vi "HFRR ADV v01.vi"() -> ()   [LabVIEW 2025] (continued)
      frame "Custom" {
      }
    }
    n2158 = Or(x=w2405, y=w2403) -> (x .or. y?=w2404:bool)
    n2159 = case shown="\"About\"" w2402 {
      tunnel: [T29."Acquire" ("Main Tab") T29."Compare Files" ("Main Tab") T29."About" ("Main Tab")] -> w2413
      frame "Acquire", Default {
      }
      frame "Compare Files" {
      }
      frame "About" {
      }
    }
    n2160 = Or(x=w2408, y="OPEN") -> (x .or. y?=w2409:bool)
    n2161 = case shown="True" w2409 {
      tunnel: w2408 -> [_ w2441]
      frame False {
      }
      frame True {
        n2162 = stacked-sequence {
          tunnel: w2441 -> [_ w2508 _ _]
          frame #0 {
            w2457 = "  " ("String 6")
            n2163 = local write "OPEN"(FALSE ("open")) -> ()
            n2164 = local read "string1 2"() -> (w2445:string)
            n2165 = local read "string1 3"() -> (w2444:string)
            n2166 = local read "string1 4"() -> (w2443:string)
            n2167 = property on="OPEN" class="Bool (strict)"("Visible"=FALSE) -> ()  [unwired: 2 in, 2 out]
            n2168 = local write "String 6"(w2457) -> ()
            n2169 = local write "String 7"(w2457) -> ()
            n2170 = local write "String 8"(w2457) -> ()
            n2171 = local write "String 12"(w2457) -> ()
            n2172 = local read "OK Button 16"() -> (w2442:bool)
            n2173 = String To Path(string=w2445) -> (path=w2453:path)
            n2174 = String To Path(string=w2444) -> (path=w2452:path)
            n2175 = String To Path(string=w2443) -> (path=w2451:path)
            n2176 = case shown="True" w2442 {
              tunnel: [w2458 w2459] -> w2446
              frame False {
                n2177 = local read "string1"() -> (w2458:string)
              }
              frame True {
                n2178 = local read "String Indicator 4"() -> (w2459:string)
              }
            }
            n2179 = Open/Create/Replace File "Open File"(file path (use dialog)=w2453) -> (refnum out=w2449:refnum<file>)  [unwired: 5 in, 2 out]
            n2180 = Open/Create/Replace File "Open File"(file path (use dialog)=w2452) -> (refnum out=w2448:refnum<file>)  [unwired: 5 in, 2 out]
            n2181 = Open/Create/Replace File "Open File"(file path (use dialog)=w2451) -> (refnum out=w2447:refnum<file>)  [unwired: 5 in, 2 out]
            n2182 = while {
              tunnel: w2449 -> [w2471]
              i -> [w2467]
              stop <- w2466 continue-if-true
              (unwired) TRUE ("line mode (F)")
              n2183 = Read from Text File "Read File"(file (use dialog)=w2471) -> (text=w2468:string)  [unwired: 3 in, 3 out]
              n2184 = local write "Numeric 11"(w2467) -> ()
              n2185 = String Length(string=w2468) -> (length=w2470:i32)
              n2186 = Greater?(x=w2470, y=1) -> (0:w2466:bool)
            }
            n2187 = while {
              tunnel: w2448 -> [w2477]
              i -> [w2473]
              stop <- w2472 continue-if-true
              (unwired) TRUE ("line mode (F)")
              n2188 = Read from Text File "Read File"(file (use dialog)=w2477) -> (text=w2474:string)  [unwired: 3 in, 3 out]
              n2189 = local write "Numeric 12"(w2473) -> ()
              n2190 = String Length(string=w2474) -> (length=w2476:i32)
              n2191 = Greater?(x=w2476, y=1) -> (0:w2472:bool)
            }
            n2192 = while {
              tunnel: w2447 -> [w2483]
              i -> [w2479]
              stop <- w2478 continue-if-true
              (unwired) TRUE ("line mode (F)")
              n2193 = Read from Text File "Read File"(file (use dialog)=w2483) -> (text=w2480:string)  [unwired: 3 in, 3 out]
              n2194 = local write "Numeric 13"(w2479) -> ()
              n2195 = String Length(string=w2480) -> (length=w2482:i32)
              n2196 = Greater?(x=w2482, y=1) -> (0:w2478:bool)
            }
            n2197 = String To Path(string=w2446) -> (path=w2454:path)
            n2198 = Open/Create/Replace File "Open File"(file path (use dialog)=w2454) -> (refnum out=w2450:refnum<file>)  [unwired: 5 in, 2 out]
            n2199 = while {
              tunnel: w2450 -> [w2465]
              i -> [w2461]
              stop <- w2460 continue-if-true
              (unwired) TRUE ("line mode (F)")
              n2200 = Read from Text File "Read File"(file (use dialog)=w2465) -> (text=w2462:string)  [unwired: 3 in, 3 out]
              n2201 = local write "Numeric 8"(w2461) -> ()
              n2202 = String Length(string=w2462) -> (length=w2464:i32)
              n2203 = Greater?(x=w2464, y=1) -> (0:w2460:bool)
            }
          }
          frame #1 {
            w2635 = FALSE ("ACTUAL   MERGE")
            # "Sample Temp"
            # "ECR"
            # "COF"
            # "Time\nCOF\nFF\nTemp"
            n2204 = case shown="True" w2508 {
              tunnel: [w2655 w2656] -> w2509
              frame False {
                n2205 = local read "string1"() -> (w2655:string)
              }
              frame True {
                n2206 = local read "String Indicator 4"() -> (w2656:string)
              }
            }
            n2207 = local read "string1 3"() -> (w2553:string)
            n2208 = String To Path(string=w2509) -> (path=w2640:path)
            n2209 = String To Path(string=w2553) -> (path=w2651:path)
            n2210 = local read "Numeric 12"() -> (w2637:i32)
            n2211 = local read "Numeric 8"() -> (w2639:i32)
            n2212 = local read "string1 2"() -> (w2554:string)
            n2213 = local read "string1 4"() -> (w2552:string)
            n2214 = Open/Create/Replace File "Open File"(file path (use dialog)=w2640) -> (refnum out=w2654:refnum<file>, error out=w2653:errorcluster)  [unwired: 5 in, 1 out]
            n2215 = Open/Create/Replace File "Open File"(file path (use dialog)=w2651) -> (refnum out=w2647:refnum<file>, error out=w2648:errorcluster)  [unwired: 5 in, 1 out]
            n2216 = for {
              N: w2639 -> [_]
              tunnel: w2654 -> [w2802]
              tunnel: w2653 -> [w2801]
              tunnel: [w2791] -> w2566 mode=indexing
              tunnel: [w2789] -> w2623 mode=indexing
              tunnel: [w2790] -> w2618 mode=indexing
              tunnel: w2635 -> [_]
              tunnel: [w2783] -> w2620 mode=indexing
              tunnel: [w2779] -> w2589 mode=indexing
              tunnel: [w2775] -> w2564 mode=indexing
              tunnel: [w2771] -> w2545 mode=indexing
              tunnel: [w2766] -> w2505 mode=indexing
              (unwired) TRUE ("line mode (F)")
              # "freq"
              # "Stroke"
              # "Time"
              # "CoF"
              # "Humidity"
              # "Temp"
              # "Air Temp"
              # "ECR"
              n2217 = Read from Text File "Read File"(file (use dialog)=w2802, error in=w2801) -> (text=w2767:string)  [unwired: 2 in, 3 out]
              n2218 = local write "String 6"(w2767) -> ()
              n2219 = String Subset(string=w2767, offset (0)=0, length (rest)=14 ("length (rest)")) -> (substring=w2795:string)
              n2220 = String Subset(string=w2767, offset (0)=35, length (rest)=9 ("length (rest)")) -> (substring=w2792:string)
              n2221 = String Subset(string=w2767, offset (0)=15, length (rest)=9 ("length (rest)")) -> (substring=w2798:string)
              n2222 = Fract/Exp String To Number(string=w2795) -> (number=w2791:dbl)  [unwired: 3 in, 1 out]
              n2223 = Fract/Exp String To Number(string=w2792) -> (number=w2790:dbl)  [unwired: 3 in, 1 out]
              n2224 = Fract/Exp String To Number(string=w2798) -> (number=w2789:dbl)  [unwired: 3 in, 1 out]
              n2225 = String Subset(string=w2767, offset (0)=85, length (rest)=9 ("length (rest)")) -> (substring=w2768:string)
              n2226 = String Subset(string=w2767, offset (0)=25, length (rest)=9 ("length (rest)")) -> (substring=w2774:string)
              n2227 = String Subset(string=w2767, offset (0)=55, length (rest)=9 ("length (rest)")) -> (substring=w2776:string)
              n2228 = String Subset(string=w2767, offset (0)=45, length (rest)=9 ("length (rest)")) -> (substring=w2782:string)
              n2229 = String Subset(string=w2767, offset (0)=65, length (rest)=9 ("length (rest)")) -> (substring=w2788:string)
              n2230 = Fract/Exp String To Number(string=w2774) -> (number=w2771:dbl)  [unwired: 3 in, 1 out]
              n2231 = Fract/Exp String To Number(string=w2768) -> (number=w2766:dbl)  [unwired: 3 in, 1 out]
              n2232 = Fract/Exp String To Number(string=w2776) -> (number=w2775:dbl)  [unwired: 3 in, 1 out]
              n2233 = Fract/Exp String To Number(string=w2782) -> (number=w2779:dbl)  [unwired: 3 in, 1 out]
              n2234 = Fract/Exp String To Number(string=w2788) -> (number=w2785:dbl)  [unwired: 3 in, 1 out]
              n2235 = Add(x=w2785, y=0.0) -> (x+y=w2783:dbl)
            }
            n2236 = for {
              N: w2637 -> [_]
              tunnel: w2648 -> [w2728]
              tunnel: w2647 -> [w2727]
              tunnel: [w2717] -> w2606 mode=indexing
              tunnel: [w2715] -> w2604 mode=indexing
              tunnel: [w2716] -> w2600 mode=indexing
              tunnel: w2635 -> [_]
              tunnel: [w2709] -> w2602 mode=indexing
              tunnel: [w2705] -> w2584 mode=indexing
              tunnel: [w2701] -> w2560 mode=indexing
              tunnel: [w2698] -> w2541 mode=indexing
              tunnel: [w2694] -> w2500 mode=indexing
              (unwired) 9 ("length (rest)")
              (unwired) 9 ("length (rest)")
              (unwired) TRUE ("line mode (F)")
              n2237 = Read from Text File "Read File"(file (use dialog)=w2727, error in=w2728) -> (text=w2695:string)  [unwired: 2 in, 3 out]
              n2238 = local write "String 8"(w2695) -> ()
              n2239 = String Subset(string=w2695, offset (0)=85) -> (substring=w2697:string)  [unwired: 1 in]
              n2240 = String Subset(string=w2695, offset (0)=35, length (rest)=9 ("length (rest)")) -> (substring=w2718:string)
              n2241 = String Subset(string=w2695, offset (0)=55, length (rest)=9 ("length (rest)")) -> (substring=w2703:string)
              n2242 = String Subset(string=w2695, offset (0)=25) -> (substring=w2699:string)  [unwired: 1 in]
              n2243 = String Subset(string=w2695, offset (0)=15, length (rest)=9 ("length (rest)")) -> (substring=w2724:string)
              n2244 = String Subset(string=w2695, offset (0)=0, length (rest)=14 ("length (rest)")) -> (substring=w2721:string)
              n2245 = String Subset(string=w2695, offset (0)=45, length (rest)=9 ("length (rest)")) -> (substring=w2708:string)
              n2246 = String Subset(string=w2695, offset (0)=65, length (rest)=9 ("length (rest)")) -> (substring=w2714:string)
              n2247 = Fract/Exp String To Number(string=w2697) -> (number=w2694:dbl)  [unwired: 3 in, 1 out]
              n2248 = Fract/Exp String To Number(string=w2718) -> (number=w2716:dbl)  [unwired: 3 in, 1 out]
              n2249 = Fract/Exp String To Number(string=w2703) -> (number=w2701:dbl)  [unwired: 3 in, 1 out]
              n2250 = Fract/Exp String To Number(string=w2699) -> (number=w2698:dbl)  [unwired: 3 in, 1 out]
              n2251 = Fract/Exp String To Number(string=w2724) -> (number=w2715:dbl)  [unwired: 3 in, 1 out]
              n2252 = Fract/Exp String To Number(string=w2721) -> (number=w2717:dbl)  [unwired: 3 in, 1 out]
              n2253 = Fract/Exp String To Number(string=w2708) -> (number=w2705:dbl)  [unwired: 3 in, 1 out]
              n2254 = Fract/Exp String To Number(string=w2714) -> (number=w2711:dbl)  [unwired: 3 in, 1 out]
              n2255 = Add(x=w2711, y=0.0) -> (x+y=w2709:dbl)
            }
            n2256 = String To Path(string=w2554) -> (path=w2652:path)
            n2257 = String To Path(string=w2552) -> (path=w2646:path)
            n2258 = local read "Numeric 11"() -> (w2636:i32)
            n2259 = local read "Numeric 13"() -> (w2638:i32)
            n2260 = Open/Create/Replace File "Open File"(file path (use dialog)=w2652) -> (refnum out=w2650:refnum<file>, error out=w2649:errorcluster)  [unwired: 5 in, 1 out]
            n2261 = Open/Create/Replace File "Open File"(file path (use dialog)=w2646) -> (refnum out=w2645:refnum<file>, error out=w2644:errorcluster)  [unwired: 5 in, 1 out]
            n2262 = for {
              N: w2636 -> [_]
              tunnel: w2650 -> [w2765]
              tunnel: w2649 -> [w2764]
              tunnel: [w2754] -> w2616 mode=indexing
              tunnel: [w2752] -> w2614 mode=indexing
              tunnel: [w2753] -> w2609 mode=indexing
              tunnel: w2635 -> [_]
              tunnel: [w2746] -> w2611 mode=indexing
              tunnel: [w2742] -> w2587 mode=indexing
              tunnel: [w2738] -> w2562 mode=indexing
              tunnel: [w2734] -> w2543 mode=indexing
              tunnel: [w2729] -> w2501 mode=indexing
              (unwired) TRUE ("line mode (F)")
              n2263 = Read from Text File "Read File"(file (use dialog)=w2765, error in=w2764) -> (text=w2730:string)  [unwired: 2 in, 3 out]
              n2264 = local write "String 7"(w2730) -> ()
              n2265 = String Subset(string=w2730, offset (0)=85, length (rest)=9 ("length (rest)")) -> (substring=w2733:string)
              n2266 = String Subset(string=w2730, offset (0)=35, length (rest)=9 ("length (rest)")) -> (substring=w2755:string)
              n2267 = String Subset(string=w2730, offset (0)=55, length (rest)=9 ("length (rest)")) -> (substring=w2741:string)
              n2268 = String Subset(string=w2730, offset (0)=25, length (rest)=9 ("length (rest)")) -> (substring=w2735:string)
              n2269 = String Subset(string=w2730, offset (0)=45, length (rest)=9 ("length (rest)")) -> (substring=w2743:string)
              n2270 = String Subset(string=w2730, offset (0)=0, length (rest)=14 ("length (rest)")) -> (substring=w2758:string)
              n2271 = String Subset(string=w2730, offset (0)=15, length (rest)=9 ("length (rest)")) -> (substring=w2761:string)
              n2272 = String Subset(string=w2730, offset (0)=65, length (rest)=9 ("length (rest)")) -> (substring=w2747:string)
              n2273 = Fract/Exp String To Number(string=w2733) -> (number=w2729:dbl)  [unwired: 3 in, 1 out]
              n2274 = Fract/Exp String To Number(string=w2755) -> (number=w2753:dbl)  [unwired: 3 in, 1 out]
              n2275 = Fract/Exp String To Number(string=w2741) -> (number=w2738:dbl)  [unwired: 3 in, 1 out]
              n2276 = Fract/Exp String To Number(string=w2735) -> (number=w2734:dbl)  [unwired: 3 in, 1 out]
              n2277 = Fract/Exp String To Number(string=w2743) -> (number=w2742:dbl)  [unwired: 3 in, 1 out]
              n2278 = Fract/Exp String To Number(string=w2758) -> (number=w2754:dbl)  [unwired: 3 in, 1 out]
              n2279 = Fract/Exp String To Number(string=w2761) -> (number=w2752:dbl)  [unwired: 3 in, 1 out]
              n2280 = Fract/Exp String To Number(string=w2747) -> (number=w2750:dbl)  [unwired: 3 in, 1 out]
              n2281 = Add(x=w2750, y=0.0) -> (x+y=w2746:dbl)
            }
            n2282 = for {
              N: w2638 -> [_]
              tunnel: w2645 -> [w2693]
              tunnel: w2644 -> [w2692]
              tunnel: [w2682] -> w2598 mode=indexing
              tunnel: [w2681] -> w2591 mode=indexing
              tunnel: w2635 -> [_]
              tunnel: [w2670] -> w2596 mode=indexing
              tunnel: [w2675] -> w2593 mode=indexing
              tunnel: [w2671] -> w2583 mode=indexing
              tunnel: [w2666] -> w2558 mode=indexing
              tunnel: [w2662] -> w2539 mode=indexing
              tunnel: [w2657] -> w2499 mode=indexing
              (unwired) 1.0 ("x")
              (unwired) TRUE ("line mode (F)")
              n2283 = Read from Text File "Read File"(file (use dialog)=w2693, error in=w2692) -> (text=w2658:string)  [unwired: 2 in, 3 out]
              n2284 = local write "String 12"(w2658) -> ()
              n2285 = String Subset(string=w2658, offset (0)=85, length (rest)=9 ("length (rest)")) -> (substring=w2660:string)
              n2286 = String Subset(string=w2658, offset (0)=35, length (rest)=9 ("length (rest)")) -> (substring=w2683:string)
              n2287 = String Subset(string=w2658, offset (0)=55, length (rest)=9 ("length (rest)")) -> (substring=w2668:string)
              n2288 = String Subset(string=w2658, offset (0)=25, length (rest)=9 ("length (rest)")) -> (substring=w2664:string)
              n2289 = String Subset(string=w2658, offset (0)=45, length (rest)=9 ("length (rest)")) -> (substring=w2673:string)
              n2290 = String Subset(string=w2658, offset (0)=15, length (rest)=9 ("length (rest)")) -> (substring=w2689:string)
              n2291 = String Subset(string=w2658, offset (0)=0, length (rest)=14 ("length (rest)")) -> (substring=w2686:string)
              n2292 = String Subset(string=w2658, offset (0)=65, length (rest)=9 ("length (rest)")) -> (substring=w2676:string)
              n2293 = Fract/Exp String To Number(string=w2660) -> (number=w2657:dbl)  [unwired: 3 in, 1 out]
              n2294 = Fract/Exp String To Number(string=w2683) -> (number=w2681:dbl)  [unwired: 3 in, 1 out]
              n2295 = Fract/Exp String To Number(string=w2668) -> (number=w2666:dbl)  [unwired: 3 in, 1 out]
              n2296 = Fract/Exp String To Number(string=w2664) -> (number=w2662:dbl)  [unwired: 3 in, 1 out]
              n2297 = Fract/Exp String To Number(string=w2673) -> (number=w2671:dbl)  [unwired: 3 in, 1 out]
              n2298 = Fract/Exp String To Number(string=w2689) -> (number=w2670:dbl)  [unwired: 3 in, 1 out]
              n2299 = Fract/Exp String To Number(string=w2686) -> (number=w2682:dbl)  [unwired: 3 in, 1 out]
              n2300 = Fract/Exp String To Number(string=w2676) -> (number=w2679:dbl)  [unwired: 3 in, 1 out]
              n2301 = Add(x=w2679, y=0.0) -> (x+y=w2675:dbl)
            }
            n2302 = Delete From Array(array=w2541, index=0) -> (array with subset deleted=w2514:dbl[])  [unwired: 1 in, 1 out]
            n2303 = Delete From Array(array=w2604, index=0) -> (array with subset deleted=w2577:dbl[])  [unwired: 1 in, 1 out]
            n2304 = Delete From Array(array=w2584, index=0) -> (array with subset deleted=w2572:dbl[])  [unwired: 1 in, 1 out]
            n2305 = Delete From Array(array=w2602, index=0) -> (array with subset deleted=w2603:dbl[])  [unwired: 1 in, 1 out]
            n2306 = call-poly <vilib>:"Mean.vi"("X"=w2514) -> ("mean"=→"КОФ2 4":dbl)  [unwired: 1 out]
            n2307 = call-poly <vilib>:"Mean.vi"("X"=w2577) -> ("mean"=→"КОФ3":dbl)  [unwired: 1 out]
            n2308 = call-poly <vilib>:"Mean.vi"("X"=w2572) -> ("mean"=→"CP3":dbl)  [unwired: 1 out]
            n2309 = Delete From Array(array=w2566, index=0) -> (array with subset deleted=w2493:dbl[])  [unwired: 1 in, 1 out]
            n2310 = Delete From Array(array=w2505, index=0) -> (array with subset deleted=w2492:dbl[])  [unwired: 1 in, 1 out]
            n2311 = Delete From Array(array=w2545, index=0) -> (array with subset deleted=w2516:dbl[])  [unwired: 1 in, 1 out]
            n2312 = Delete From Array(array=w2623, index=0) -> (array with subset deleted=w2578:dbl[])  [unwired: 1 in, 1 out]
            n2313 = Delete From Array(array=w2589, index=0) -> (array with subset deleted=w2574:dbl[])  [unwired: 1 in, 1 out]
            "array w/ subset deleted" <- w2574
            n2314 = Delete From Array(array=w2620, index=0) -> (array with subset deleted=w2621:dbl[])  [unwired: 1 in, 1 out]
            n2315 = call-poly <vilib>:"Mean.vi"("X"=w2516) -> ("mean"=→"КОФ2 2":dbl)  [unwired: 1 out]
            n2316 = call-poly <vilib>:"Mean.vi"("X"=w2578) -> ("mean"=→"КОФ1":dbl)  [unwired: 1 out]
            n2317 = Bundle "Bundle"(w2493, w2492) -> (w2498:cluster{dbl[], dbl[]})  [unwired: 1 in]
            n2318 = Bundle "Bundle"(w2493, w2621) -> (w2485:cluster{dbl[], dbl[]})  [unwired: 1 in]
            n2319 = Delete From Array(array=w2500, index=0) -> (array with subset deleted=w2488:dbl[])  [unwired: 1 in, 1 out]
            n2320 = Delete From Array(array=w2501, index=0) -> (array with subset deleted=w2490:dbl[])  [unwired: 1 in, 1 out]
            n2321 = Delete From Array(array=w2611, index=0) -> (array with subset deleted=w2612:dbl[])  [unwired: 1 in, 1 out]
            n2322 = Delete From Array(array=w2499, index=0) -> (array with subset deleted=w2486:dbl[])  [unwired: 1 in, 1 out]
            n2323 = Delete From Array(array=w2593, index=0) -> (array with subset deleted=w2594:dbl[])  [unwired: 1 in, 1 out]
            n2324 = Delete From Array(array=w2618, index=0) -> (array with subset deleted=w2524:dbl[])  [unwired: 1 in, 1 out]
            n2325 = Delete From Array(array=w2564, index=0) -> (array with subset deleted=w2520:dbl[])  [unwired: 1 in, 1 out]
            n2326 = Delete From Array(array=w2600, index=0) -> (array with subset deleted=w2522:dbl[])  [unwired: 1 in, 1 out]
            n2327 = Delete From Array(array=w2560, index=0) -> (array with subset deleted=w2518:dbl[])  [unwired: 1 in, 1 out]
            n2328 = Delete From Array(array=w2609, index=0) -> (array with subset deleted=w2523:dbl[])  [unwired: 1 in, 1 out]
            n2329 = Delete From Array(array=w2562, index=0) -> (array with subset deleted=w2519:dbl[])  [unwired: 1 in, 1 out]
            n2330 = Delete From Array(array=w2543, index=0) -> (array with subset deleted=w2515:dbl[])  [unwired: 1 in, 1 out]
            n2331 = Delete From Array(array=w2587, index=0) -> (array with subset deleted=w2573:dbl[])  [unwired: 1 in, 1 out]
            n2332 = Delete From Array(array=w2614, index=0) -> (array with subset deleted=w2575:dbl[])  [unwired: 1 in, 1 out]
            n2333 = Delete From Array(array=w2591, index=0) -> (array with subset deleted=w2521:dbl[])  [unwired: 1 in, 1 out]
            n2334 = Delete From Array(array=w2558, index=0) -> (array with subset deleted=w2517:dbl[])  [unwired: 1 in, 1 out]
            n2335 = Delete From Array(array=w2539, index=0) -> (array with subset deleted=w2513:dbl[])  [unwired: 1 in, 1 out]
            n2336 = Delete From Array(array=w2583, index=0) -> (array with subset deleted=w2571:dbl[])  [unwired: 1 in, 1 out]
            n2337 = Delete From Array(array=w2596, index=0) -> (array with subset deleted=w2576:dbl[])  [unwired: 1 in, 1 out]
            n2338 = Delete From Array(array=w2606, index=0) -> (array with subset deleted=w2489:dbl[])  [unwired: 1 in, 1 out]
            n2339 = Delete From Array(array=w2616, index=0) -> (array with subset deleted=w2491:dbl[])  [unwired: 1 in, 1 out]
            n2340 = Delete From Array(array=w2598, index=0) -> (array with subset deleted=w2487:dbl[])  [unwired: 1 in, 1 out]
            n2341 = Bundle "Bundle"(w2493, w2524) -> (w2511:cluster{dbl[], dbl[]})  [unwired: 1 in]
            n2342 = Bundle "Bundle"(w2493, w2578) -> (w2512:cluster{dbl[], dbl[]})  [unwired: 1 in]
            n2343 = Bundle "Bundle"(w2524, w2520) -> (w2526:cluster{dbl[], dbl[]})  [unwired: 1 in]
            n2344 = Bundle "Bundle"(w2489, w2488) -> (w2496:cluster{dbl[], dbl[]})  [unwired: 1 in]
            n2345 = Bundle "Bundle"(w2522, w2518) -> (w2528:cluster{dbl[], dbl[]})  [unwired: 1 in]
            n2346 = Bundle "Bundle"(w2489, w2522) -> (w2632:cluster{dbl[], dbl[]})  [unwired: 1 in]
            n2347 = Bundle "Bundle"(w2489, w2518) -> (w2556:cluster{dbl[], dbl[]})  [unwired: 1 in]
            n2348 = Bundle "Bundle"(w2489, w2577) -> (w2642:cluster{dbl[], dbl[]})  [unwired: 1 in]
            n2349 = Bundle "Bundle"(w2489, w2572) -> (w2580:cluster{dbl[], dbl[]})  [unwired: 1 in]
            n2350 = Bundle "Bundle"(w2489, w2603) -> (w2627:cluster{dbl[], dbl[]})  [unwired: 1 in]
            n2351 = Bundle "Bundle"(w2523, w2519) -> (w2527:cluster{dbl[], dbl[]})  [unwired: 1 in]
            n2352 = Bundle "Bundle"(w2491, w2490) -> (w2497:cluster{dbl[], dbl[]})  [unwired: 1 in]
            n2353 = Bundle "Bundle"(w2491, w2523) -> (w2634:cluster{dbl[], dbl[]})  [unwired: 1 in]
            n2354 = Bundle "Bundle"(w2491, w2519) -> (w2557:cluster{dbl[], dbl[]})  [unwired: 1 in]
            n2355 = Bundle "Bundle"(w2491, w2573) -> (w2581:cluster{dbl[], dbl[]})  [unwired: 1 in]
            n2356 = Bundle "Bundle"(w2491, w2575) -> (w2643:cluster{dbl[], dbl[]})  [unwired: 1 in]
            n2357 = Bundle "Bundle"(w2491, w2612) -> (w2625:cluster{dbl[], dbl[]})  [unwired: 1 in]
            n2358 = Bundle "Bundle"(w2521, w2517) -> (w2529:cluster{dbl[], dbl[]})  [unwired: 1 in]
            n2359 = Bundle "Bundle"(w2487, w2486) -> (w2495:cluster{dbl[], dbl[]})  [unwired: 1 in]
            n2360 = Bundle "Bundle"(w2487, w2521) -> (w2633:cluster{dbl[], dbl[]})  [unwired: 1 in]
            n2361 = Bundle "Bundle"(w2487, w2517) -> (w2555:cluster{dbl[], dbl[]})  [unwired: 1 in]
            n2362 = Bundle "Bundle"(w2487, w2571) -> (w2579:cluster{dbl[], dbl[]})  [unwired: 1 in]
            n2363 = Bundle "Bundle"(w2487, w2576) -> (w2641:cluster{dbl[], dbl[]})  [unwired: 1 in]
            n2364 = Bundle "Bundle"(w2487, w2594) -> (w2626:cluster{dbl[], dbl[]})  [unwired: 1 in]
            n2365 = call-poly <vilib>:"Mean.vi"("X"=w2574) -> ("mean"=→"CP1":dbl)  [unwired: 1 out]
            n2366 = call-poly <vilib>:"Mean.vi"("X"=w2515) -> ("mean"=→"КОФ2 3":dbl)  [unwired: 1 out]
            n2367 = call-poly <vilib>:"Mean.vi"("X"=w2573) -> ("mean"=→"CP2":dbl)  [unwired: 1 out]
            n2368 = call-poly <vilib>:"Mean.vi"("X"=w2575) -> ("mean"=→"КОФ2":dbl)  [unwired: 1 out]
            n2369 = call-poly <vilib>:"Mean.vi"("X"=w2513) -> ("mean"=→"КОФ2 5":dbl)  [unwired: 1 out]
            n2370 = call-poly <vilib>:"Mean.vi"("X"=w2571) -> ("mean"=→"CP4":dbl)  [unwired: 1 out]
            n2371 = call-poly <vilib>:"Mean.vi"("X"=w2576) -> ("mean"=→"КОФ4":dbl)  [unwired: 1 out]
            n2372 = Bundle "Bundle"(w2493, w2520) -> (w2484:cluster{dbl[], dbl[]})  [unwired: 1 in]
            n2373 = Bundle "Bundle"(w2493, w2574) -> (w2507:cluster{dbl[], dbl[]})  [unwired: 1 in]
            n2374 = Build Array "Build Array"(w2484, w2507) -> (w2510:cluster{dbl[], dbl[]}[])
            "XY Graph 17" <- w2510
            n2375 = Build Array "Build Array"(w2498, w2497, w2496, w2495) -> (→"Frequency ( Hz )":cluster{dbl[], dbl[]}[])
            n2376 = Build Array "Build Array"(w2526, w2527, w2528, w2529) -> (→"Air Temp ( °C ) vs Humidity ( % RH )":cluster{dbl[], dbl[]}[])
            n2377 = Build Array "Build Array"(w2511, w2634, w2632, w2633) -> (→"Air Temperature  ( °C )":cluster{dbl[], dbl[]}[])
            n2378 = Build Array "Build Array"(w2484, w2557, w2556, w2555) -> (→"Humidity ( %RH )":cluster{dbl[], dbl[]}[])
            n2379 = Build Array "Build Array"(w2512, w2643, w2642, w2641) -> (→"Coefficient Of Friction":cluster{dbl[], dbl[]}[])
            n2380 = Build Array "Build Array"(w2507, w2581, w2580, w2579) -> (→"Sample Temperature ( °C )":cluster{dbl[], dbl[]}[])
            n2381 = Build Array "Build Array"(w2485, w2625, w2627, w2626) -> (→"XY Graph 13":cluster{dbl[], dbl[]}[])
            n2382 = Bundle "Bundle"(w2493, w2516) -> (w2538:cluster{dbl[], dbl[]})  [unwired: 1 in]
            n2383 = Bundle "Bundle"(w2489, w2514) -> (w2536:cluster{dbl[], dbl[]})  [unwired: 1 in]
            n2384 = Bundle "Bundle"(w2491, w2515) -> (w2537:cluster{dbl[], dbl[]})  [unwired: 1 in]
            n2385 = Bundle "Bundle"(w2487, w2513) -> (w2535:cluster{dbl[], dbl[]})  [unwired: 1 in]
            n2386 = Build Array "Build Array"(w2538, w2537, w2536, w2535) -> (→"Stroke ( mm )":cluster{dbl[], dbl[]}[])
            n2387 = local write "XY Graph 16"(w2510) -> ()
          }
          frame #2 {
          }
          frame #3 {
            n2388 = local write "Numeric 8"(0 ("Numeric 8")) -> ()
            n2389 = local write "Numeric 11"(0 ("Numeric 11")) -> ()
            n2390 = local write "Numeric 12"(0 ("Numeric 12")) -> ()
            n2391 = local write "Numeric 13"(0 ("Numeric 13")) -> ()
            n2392 = property on="OPEN" class="Bool (strict)"("Visible"=TRUE) -> ()  [unwired: 2 in, 2 out]
            n2393 = local read "String Control 2"() -> (w2810:string)
            n2394 = local read "String Control 4"() -> (w2809:string)
            n2395 = local read "String Control 6"() -> (w2808:string)
            n2396 = local read "String Control 8"() -> (w2807:string)
            n2397 = Match Pattern(string=w2810, regular expression="Samples / cycle :- ") -> (after substring=w2824:string)  [unwired: 1 in, 3 out]
            n2398 = Match Pattern(string=w2810, regular expression="Frequency :- ") -> (after substring=w2843:string)  [unwired: 1 in, 3 out]
            n2399 = Match Pattern(string=w2809, regular expression="Samples / cycle :- ") -> (after substring=w2820:string)  [unwired: 1 in, 3 out]
            n2400 = Match Pattern(string=w2809, regular expression="Frequency :- ") -> (after substring=w2838:string)  [unwired: 1 in, 3 out]
            n2401 = Match Pattern(string=w2808, regular expression="Samples / cycle :- ") -> (after substring=w2816:string)  [unwired: 1 in, 3 out]
            n2402 = Match Pattern(string=w2808, regular expression="Frequency :- ") -> (after substring=w2833:string)  [unwired: 1 in, 3 out]
            n2403 = Match Pattern(string=w2807, regular expression="Samples / cycle :- ") -> (after substring=w2812:string)  [unwired: 1 in, 3 out]
            n2404 = Match Pattern(string=w2807, regular expression="Frequency :- ") -> (after substring=w2828:string)  [unwired: 1 in, 3 out]
            n2405 = String Subset(string=w2824, length (rest)=6 ("length (rest)")) -> (substring=w2826:string)  [unwired: 1 in]
            n2406 = String Subset(string=w2843, length (rest)=9 ("length (rest)")) -> (substring=w2845:string)  [unwired: 1 in]
            n2407 = String Subset(string=w2820, length (rest)=6 ("length (rest)")) -> (substring=w2822:string)  [unwired: 1 in]
            n2408 = String Subset(string=w2838, length (rest)=9 ("length (rest)")) -> (substring=w2840:string)  [unwired: 1 in]
            n2409 = String Subset(string=w2816, length (rest)=6 ("length (rest)")) -> (substring=w2818:string)  [unwired: 1 in]
            n2410 = String Subset(string=w2833, length (rest)=9 ("length (rest)")) -> (substring=w2835:string)  [unwired: 1 in]
            n2411 = String Subset(string=w2812, length (rest)=6 ("length (rest)")) -> (substring=w2814:string)  [unwired: 1 in]
            n2412 = String Subset(string=w2828, length (rest)=9 ("length (rest)")) -> (substring=w2830:string)  [unwired: 1 in]
            n2413 = Fract/Exp String To Number(string=w2826) -> (number=w2806:dbl)  [unwired: 3 in, 1 out]
            n2414 = Fract/Exp String To Number(string=w2845) -> (number=w2846:dbl)  [unwired: 3 in, 1 out]
            n2415 = Fract/Exp String To Number(string=w2822) -> (number=w2805:dbl)  [unwired: 3 in, 1 out]
            n2416 = Fract/Exp String To Number(string=w2840) -> (number=w2841:dbl)  [unwired: 3 in, 1 out]
            n2417 = Fract/Exp String To Number(string=w2818) -> (number=w2804:dbl)  [unwired: 3 in, 1 out]
            n2418 = Fract/Exp String To Number(string=w2835) -> (number=w2836:dbl)  [unwired: 3 in, 1 out]
            n2419 = Fract/Exp String To Number(string=w2814) -> (number=w2803:dbl)  [unwired: 3 in, 1 out]
            n2420 = Fract/Exp String To Number(string=w2830) -> (number=w2831:dbl)  [unwired: 3 in, 1 out]
            n2421 = local write "sample1"(w2806) -> ()
            n2422 = local write "freq1"(w2846) -> ()
            n2423 = local write "sample2"(w2805) -> ()
            n2424 = local write "freq2"(w2841) -> ()
            n2425 = local write "sample3"(w2804) -> ()
            n2426 = local write "freq3"(w2836) -> ()
            n2427 = local write "sample4"(w2803) -> ()
            n2428 = local write "freq 4"(w2831) -> ()
          }
        }
      }
    }
    n2429 = case shown="True" w2404 {
      selector: w2404 -> [_ w2423]
      frame False {
      }
      frame True {
        n2430 = Not(x=w2423) -> (.not. x?=w2419:bool)
        n2431 = local write "service 3"(w2419) -> ()
        n2432 = local write "OPEN 6"(w2419) -> ()
        n2433 = call <vilib>:"System Exec.vi"("wait until completion? (T)"=TRUE, "command line"="C:\\LAB-IQ\\Scar View.exe") -> ("error out"=→"error out 5":errorcluster)  [unwired: 6 in, 3 out]
      }
    }
    n2434 = case shown="\"Acquire\", Default" w2413 {
      frame "Acquire", Default {
        # "Elapsed time\ncof\nstroke\nAir temp\nTemp\nHumidity"
        n2435 = disable-structure shown="Disabled" {
          frame Disabled {
            n2436 = local read "Flag"() -> (w3130:dbl)
            n2437 = local read "RUN"() -> (w3127:bool)
            n2438 = Not(x=w3127) -> (.not. x?=w3126:bool)
            n2439 = Equal?(x=w3130, y=10.0) -> (x = y?=w3128:bool)
            n2440 = And(x=w3128, y=w3126) -> (x .and. y?=w3125:bool)
            n2441 = case shown="True" w3125 {
              frame False {
              }
              frame True {
                w3131 = FALSE ("Heater Button")
                n2442 = local write "Humidity"(w3131) -> ()
                n2443 = local write "Heater Button"(w3131) -> ()
              }
            }
          }
          frame Enabled {
          }
        }
        n2444 = local read "DEMO"() -> (w3108:bool)
        n2445 = disable-structure shown="Disabled" {
          frame Disabled {
            n2446 = case shown="True" {
              selector: _ -> [_ _]
              frame False {
              }
              frame True {
                w3176 = TRUE ("Heater")
                n2447 = local write "Humidity"(w3176) -> ()
                n2448 = local write "Heater Button"(w3176) -> ()
                n2449 = local read "TEST STANDARD"() -> (w3179:T5)
                n2450 = local read "TEST STANDARD"() -> (w3174:T5)
                n2451 = Equal?(x=w3179, y=enum16{"ASTM D6079", "ISO 12156", "Custom"}."ISO 12156" ("Test Standard")) -> (x = y?=w3177:bool)
                n2452 = Equal?(x=w3174, y=enum16{"ASTM D6079", "ISO 12156", "Custom"}."ASTM D6079" ("Test Standard")) -> (x = y?=w3173:bool)
                n2453 = case shown="True" w3177 {
                  frame False {
                  }
                  frame True {
                    n2454 = local write "airtempflg"(FALSE ("airtempflg")) -> ()
                    n2455 = local write item#-1(TRUE ("Heater")) -> ()
                  }
                }
                n2456 = case shown="True" w3173 {
                  frame False {
                  }
                  frame True {
                    n2457 = local write "airtempflg"(TRUE ("airtempflg")) -> ()
                    n2458 = local write item#-1(FALSE ("Heater")) -> ()
                  }
                }
              }
            }
          }
          frame Enabled {
          }
        }
        n2459 = stacked-sequence {
          frame #0 {
            n2460 = case shown="True" "RST FF" {
              frame False {
              }
              frame True {
                w3193 = 0.0 ("X Scale.Range:Maximum")
                n2461 = property on="Frictional Force ( N )" class="WFChart (strict)"("XScale.Maximum"=600.0 ("X Scale.Range:Maximum"), "XScale.Minimum"=w3193, "YScale.Maximum"=10.0 ("Y Scale.Range:Maximum"), "YScale.Minimum"=w3193) -> ()  [unwired: 2 in, 2 out]
              }
            }
          }
          frame #1 {
            n2462 = case shown="True" "RST TEMP" {
              frame False {
              }
              frame True {
                n2463 = property on="Temperature ( Deg C )" class="WFChart (strict)"("XScale.Minimum"=0.0 ("X Scale.Range:Minimum"), "XScale.Maximum"=600.0 ("X Scale.Range:Maximum"), "YScale.Minimum"=0.0 ("Y Scale.Range:Minimum"), "YScale.Maximum"=100.0 ("Y Scale.Range:Maximum")) -> ()  [unwired: 2 in, 2 out]
              }
            }
          }
          frame #2 {
            n2464 = case shown="True" "RSTCOF" {
              frame False {
              }
              frame True {
                n2465 = property on="Coefficient of Friction" class="WFChart (strict)"("XScale.Minimum"=0.0 ("X Scale.Range:Minimum"), "XScale.Maximum"=600.0 ("X Scale.Range:Maximum"), "YScale.Maximum"=1.0 ("X Scale.Range:Minimum"), "YScale.Minimum"=0.0 ("X Scale.Range:Minimum")) -> ()  [unwired: 2 in, 2 out]
              }
            }
          }
          frame #3 {
            n2466 = case shown="True" "RSTCOF 2" {
              frame False {
              }
              frame True {
                (unwired) 100.0 ("Y Scale.Range:Maximum")
                (unwired) 0.0 ("Y Scale.Range:Minimum")
                (unwired) 600.0 ("X Scale.Range:Maximum")
                (unwired) 0.0 ("X Scale.Range:Minimum")
              }
            }
          }
          frame #4 {
            n2467 = case shown="True" "RSTCOF 3" {
              frame False {
              }
              frame True {
                n2468 = property on="Electrical Contact Resistance ( % )" class="WFChart (strict)"("XScale.Minimum"=0.0 ("X Scale.Range:Minimum"), "XScale.Maximum"=600.0 ("X Scale.Range:Maximum"), "YScale.Minimum"=0.0 ("Y Scale.Range:Minimum"), "YScale.Maximum"=100.0 ("Y Scale.Range:Maximum")) -> ()  [unwired: 2 in, 2 out]
              }
            }
          }
        }
        n2469 = local read "RUN"() -> (w3113:bool)
        n2470 = case shown="False" w3113 {
          frame False {
          }
          frame True {
          }
        }
        n2471 = case shown="False" w3108 {
          tunnel: [w3117 TRUE ("TEST RUNNING")] -> w3116
          frame False {
            n2472 = local read "RUN"() -> (w3118:bool)
            n2473 = case shown="False" w3118 {
              tunnel: [FALSE ("TEST RUNNING") TRUE ("TEST RUNNING")] -> w3117
              frame False {
                w3119 = 0.0 ("Flag")
                n2474 = local write "Elapsed time"(0.0 ("elapsedtime")) -> ()
                n2475 = local write "Time Remaining"(w3119) -> ()
                n2476 = local write "Flag"(w3119) -> ()
                n2477 = local write "Remaining Time"(w3119) -> ()
              }
              frame True {
                n2478 = local write "Flag"(10.0 ("Flag")) -> ()
              }
            }
          }
          frame True {
          }
        }
        n2479 = local read "Main Tab"() -> (w3110:T4)
        n2480 = local read "AIR TEMP"() -> (w3111:dbl)
        n2481 = Greater Or Equal?(x=w3111, y=15.0) -> (x >= y?=w3112:bool)
        "powstat" <- w3112
        n2482 = case shown="True" "Save & Continue" {
          frame False {
          }
          frame True {
            n2483 = local read "USER ID"() -> (w3518:string)
            n2484 = local read "FILE"() -> (w3526:string)
            n2485 = String Length(string=w3526) -> (length=w3524:i32)
            n2486 = String Length(string=w3518) -> (length=w3521:i32)
            n2487 = Greater?(x=w3524, y=0) -> (0:w3523:bool)
            n2488 = Greater?(x=w3521, y=0) -> (0:w3520:bool)
            n2489 = And(x=w3523, y=w3520) -> (x .and. y?=w3519:bool)
            n2490 = case shown="True" w3519 {
              frame False {
                n2491 = stacked-sequence {
                  frame #0 {
                    n2492 = One Button Dialog(message="Please Enter a File Name and Operator ID to save data !", button name ("OK")="Ok") -> ()  [unwired: 1 out]
                  }
                  frame #1 {
                    n2493 = local write "Save & Continue"(FALSE ("OK Button")) -> ()
                  }
                }
                n2494 = local write "Save & Continue"(FALSE ("OK Button")) -> ()
              }
              frame True {
                n2495 = stacked-sequence {
                  frame #0 {
                    n2496 = local read "FILE"() -> (w3532:string)
                    n2497 = call "file check.vi"("file name in"=w3532) -> ("file name out"=w3531:string)  [unwired: 9 in, 1 out]
                    n2498 = call <vilib>:"Application Directory.vi"() -> ("Application Directory"=w3542:path)
                    n2499 = Build Path(base path=w3542, name or relative path="data") -> (appended path=w3541:path)
                    n2500 = call <vilib>:"Trim Whitespace.vi"("string"=w3531) -> ("trimmed string"=w3539:string)  [unwired: 1 in]
                    n2501 = call <vilib>:"Trim Whitespace.vi"("string"=w3531) -> ("trimmed string"=w3540:string)  [unwired: 1 in]
                    n2502 = List Folder(path=w3541) -> (folder names=w3537:string[])  [unwired: 3 in, 3 out]
                    n2503 = Match Pattern(string=w3539, regular expression="_(") -> (before substring=w3536:string)  [unwired: 1 in, 3 out]
                    n2504 = for {
                      tunnel: w3537 -> [w3551] mode=indexing
                      tunnel: w3536 -> [w3549]
                      shift-right: [w3547] -> w3534
                      shift-left: bool[] [] -> [w3548]
                      n2505 = Match Pattern(string=w3551, regular expression="_(") -> (before substring=w3550:string)  [unwired: 1 in, 3 out]
                      n2506 = Equal?(x=w3550, y=w3549) -> (x = y?=w3546:bool)
                      n2507 = case shown="True" w3546 {
                        tunnel: w3546 -> [_ w3554]
                        tunnel: w3548 -> [w3553 w3556]
                        tunnel: [w3553 w3555] -> w3547
                        frame False {
                        }
                        frame True {
                          n2508 = Insert Into Array(array=w3556, new element=w3554) -> (w3555:bool[])  [unwired: 1 in]
                        }
                      }
                    }
                    n2509 = Equal?(x=w3537, y=w3536) -> (x = y?=w3545:bool[])
                    n2510 = Or Array Elements(Boolean array=w3545) -> (logical OR=w3544:bool)
                    n2511 = Array Size(array=w3534) -> (size(s)=w3533:i32)
                    n2512 = case shown="True" w3544 {
                      tunnel: w3540 -> [_ w3564]
                      tunnel: w3533 -> [_ w3557]
                      frame False {
                      }
                      frame True {
                        n2513 = Number To Decimal String(number=w3557) -> (decimal integer string=w3560:string)  [unwired: 1 in]
                        n2514 = Search/Split String(string=w3564, search string/char (-)="_(" ("regular expression")) -> (substring before match=w3562:string)  [unwired: 1 in, 2 out]
                        n2515 = Concatenate Strings(w3562, "_(" ("regular expression"), w3560, ")" ("regular expression")) -> (w3558:string)
                        n2516 = local write "FILE"(w3558) -> ()
                      }
                    }
                  }
                  frame #1 {
                    w3567 = 0.0
                    w3580 = cluster{"y":dbl, dbl, "y":dbl}[] [] ("History Data")
                    w3581 = FALSE ("Heater Button")
                    (unwired) ")!" ("string")
                    (unwired) ")" ("string")
                    w3579 = dbl[] [] ("History Data")
                    w3585 = "\r"
                    # "C:\\WinDucom\\Data\\"
                    # "C:\\LAB-IQ-NXT\\data"
                    n2517 = local write "Humidity ( %RH )"(w3567) -> ()
                    n2518 = local write "Frequency ( Hz )"(w3567) -> ()
                    n2519 = local write "Stroke 3"(w3567) -> ()
                    n2520 = local write "speedop"(0.0 ("PIDclk 2")) -> ()
                    n2521 = local write "Set Temp 2"(65.0 ("Set Temp 2")) -> ()
                    n2522 = local write "AIR TEMP"(w3567) -> ()
                    n2523 = local write "clk"(0.0 ("clk")) -> ()
                    n2524 = local write "Stroke 4"(w3567) -> ()
                    n2525 = local write "COF 2"(w3567) -> ()
                    n2526 = local write "TEMP"(w3567) -> ()
                    n2527 = local write "ecr 3"(w3567) -> ()
                    n2528 = local write "FF 3"(w3567) -> ()
                    n2529 = local write "FF 2"(w3567) -> ()
                    n2530 = property on="Coefficient of Friction" class="WFChart (strict)"("History Data"=w3579) -> ()  [unwired: 2 in, 2 out]
                    n2531 = property on="Coefficient of Friction" class="WFChart (strict)"("History Data"=w3579) -> ()  [unwired: 2 in, 2 out]
                    n2532 = property on="Frictional Force ( N )" class="WFChart (strict)"("History Data"=w3579) -> ()  [unwired: 2 in, 2 out]
                    n2533 = property on="Electrical Contact Resistance ( % )" class="WFChart (strict)"("History Data"=w3579) -> ()  [unwired: 2 in, 2 out]
                    n2534 = property on="Electrical Contact Resistance ( % )" class="WFChart (strict)"("History Data"=w3579) -> ()  [unwired: 2 in, 2 out]
                    n2535 = property on="Temperature ( Deg C )" class="WFChart (strict)"("History Data"=w3579) -> ()  [unwired: 2 in, 2 out]
                    n2536 = property on="Frictional Force ( N )" class="WFChart (strict)"("History Data"=w3579) -> ()  [unwired: 2 in, 2 out]
                    n2537 = property on="Coefficient of Friction" class="WFChart (strict)"("History Data"=w3579) -> ()  [unwired: 2 in, 2 out]
                    n2538 = property on="Frictional Force ( N )" class="WFChart (strict)"("History Data"=w3579) -> ()  [unwired: 2 in, 2 out]
                    n2539 = property on="Electrical Contact Resistance ( % )" class="WFChart (strict)"("History Data"=w3579) -> ()  [unwired: 2 in, 2 out]
                    n2540 = property on="Temperature ( Deg C )" class="WFChart (strict)"("History Data"=w3579) -> ()  [unwired: 2 in, 2 out]
                    n2541 = property on="Stroke ( mm )" class="WFChart (strict)"("History Data"=w3580) -> ()  [unwired: 2 in, 2 out]
                    n2542 = property on="Stroke ( mm )" class="WFChart (strict)"("History Data"=w3580) -> ()  [unwired: 2 in, 2 out]
                    n2543 = local write "Humidity"(w3581) -> ()
                    n2544 = local write "Heater Button"(w3581) -> ()
                    n2545 = local read "FILE"() -> (w3575:string)
                    n2546 = disable-structure shown="Enabled" {
                      disable-tunnel: [w3619 _] -> w3566
                      frame Enabled {
                        n2547 = local read "NORMAL LOAD"() -> (w3619:dbl)
                      }
                      frame Disabled {
                      }
                    }
                    n2548 = call "file check.vi"("file name in"=w3575) -> ("error out"=w3578:errorcluster, "file name out"=w3572:string)  [unwired: 9 in]
                    n2549 = call "FILE PATH CREATION.vi"("error in"=w3578, "FILE NAME :"=w3572) -> ("FILE OUT"=w3571:path)  [unwired: 8 in, 1 out]
                    n2550 = Concatenate Strings(w3572, ".dgf" ("Substring")) -> (w3577:string)
                    n2551 = Concatenate Strings(w3572, ".duf" ("Substring")) -> (w3573:string)
                    n2552 = Multiply(x=w3566, y=1.0) -> (x*y=w3598:dbl)
                    n2553 = Build Path(base path=w3571, name or relative path=w3577) -> (appended path=w3570:path)
                    n2554 = Build Path(base path=w3571, name or relative path=w3573) -> (appended path=w3569:path)
                    n2555 = Number To Fractional String(number=w3598, width (-)=i16 5, precision (6)=i16 2) -> (F-format string=w3606:string)  [unwired: 1 in]
                    n2556 = local read "tested by"() -> (w3565:string)
                    n2557 = local read "Fuel Discription :"() -> (w3594:string)
                    n2558 = local read "Batch Ref Num :"() -> (w3583:string)
                    n2559 = Get Date/Time String(date format (0)=enum16{"short", "long", "abbreviated"}."short") -> (date string=w3617:string, time string=w3614:string)  [unwired: 2 in]
                    n2560 = local read "Remarks :"() -> (w3593:string)
                    n2561 = Concatenate Strings("Load :- " ("Substring"), w3606, " grams ," ("Substring")) -> (w3605:string)
                    n2562 = local read "String 41"() -> (w3586:string)
                    n2563 = Concatenate Strings(w3594) -> (w3595:string)
                    n2564 = Concatenate Strings(w3583) -> (w3582:string)
                    n2565 = Concatenate Strings(w3565) -> (w3589:string)
                    n2566 = Concatenate Strings("(" ("Substring"), w3617, ")" ("Substring"), w3614) -> (w3588:string)
                    "concatenated string" <- w3588
                    n2567 = Concatenate Strings(w3593, "," ("string")) -> (w3592:string)
                    n2568 = Concatenate Strings("  TIME;      COF;       STROKE;     AIR TEMP;  TEMP;  HUMIDITY;  ECR; PID-OUT; FREQUENCY" ("Substring"), "\r") -> (w3601:string)
                    n2569 = Concatenate Strings(w3586, w3585, "Fuel Discription :-" ("Substring"), w3595, w3585, w3605, w3585, "Batch Ref Num :-" ("Substring"), w3582, w3585, " Remarks :- " ("Substring"), w3592, w3585, " Date :- " ("Substring"), w3588, w3585, "Tested By :-" ("Substring"), w3589) -> (w3599:string)
                    "REMARKS" <- w3599
                    n2570 = call <vilib>:"Write Characters To File.vi"("append to file? (new file:F)"=FALSE, "character string"=w3601, "file path (dialog if empty)"=w3570) -> ()  [unwired: 2 in, 1 out]
                    n2571 = call <vilib>:"Write Characters To File.vi"("append to file? (new file:F)"=FALSE, "character string"=w3599, "file path (dialog if empty)"=w3569) -> ()  [unwired: 2 in, 1 out]
                  }
                  frame #2 {
                    n2572 = local write "Cycles elapsed"(0 ("Cycles elapsed")) -> ()
                    n2573 = local write "cyclecount"(0 ("cyclecount")) -> ()
                    n2574 = local write "Save & Continue"(FALSE ("OK")) -> ()
                    n2575 = local write "autostrtflg"(TRUE ("autostrtflg")) -> ()
                    n2576 = local write "Save"(FALSE ("Save")) -> ()
                    n2577 = Get Date/Time In Seconds() -> (seconds since 1Jan1904=w3624:timestamp)
                    n2578 = To Double Precision Float(number=w3624) -> (double precision float=w3623:dbl)
                    n2579 = local write "acq timer"(w3623) -> ()
                    n2580 = One Button Dialog(message="Please ensure sample is mounted properly and machine is ready in all aspects for testing !", button name ("OK")="Ok") -> ()  [unwired: 1 out]
                  }
                  frame #3 {
                    n2581 = stacked-sequence {
                      frame #0 {
                        n2582 = local write "Main Dashboard Buttons"(T1."Dashboard" ("Main Dashboard Buttons")) -> ()
                        n2583 = local write "Main Tab"(T4."Acquire" ("Main Tab")) -> ()
                      }
                      frame #1 {
                        n2584 = local write "EVENT LOG"("" ("EVENT LOG")) -> ()
                      }
                      frame #2 {
                        n2585 = Wait (ms)(milliseconds to wait=u32 50) -> ()  [unwired: 1 out]
                      }
                      frame #3 {
                        n2586 = disable-structure shown="Disabled" {
                          frame Disabled {
                            n2587 = local read "EVENT LOG"() -> (w3636:string)
                            n2588 = call "Event Log.vi"("Content"="Test Details", "EVENT LOG"=w3636) -> ("EVENT LOG"=w3635:string)  [unwired: 8 in, 1 out]
                            n2589 = local write "EVENT LOG"(w3635) -> ()
                          }
                          frame Enabled {
                          }
                        }
                      }
                      frame #4 {
                        n2590 = Wait (ms)(milliseconds to wait=u32 50) -> ()  [unwired: 1 out]
                      }
                      frame #5 {
                        n2591 = local read "FILE"() -> (w3638:string)
                        n2592 = Concatenate Strings("File Name :" ("Content"), w3638) -> (w3639:string)
                        n2593 = local read "EVENT LOG"() -> (w3642:string)
                        n2594 = call "Event Log.vi"("Content"=w3639, "EVENT LOG"=w3642) -> ("EVENT LOG"=w3641:string)  [unwired: 8 in, 1 out]
                        n2595 = local write "EVENT LOG"(w3641) -> ()
                      }
                      frame #6 {
                        n2596 = Wait (ms)(milliseconds to wait=u32 50) -> ()  [unwired: 1 out]
                      }
                      frame #7 {
                        n2597 = local read "Batch Ref Num :"() -> (w3644:string)
                        n2598 = Concatenate Strings("Batch Ref No :" ("Content"), w3644) -> (w3645:string)
                        n2599 = local read "EVENT LOG"() -> (w3648:string)
                        n2600 = call "Event Log.vi"("Content"=w3645, "EVENT LOG"=w3648) -> ("EVENT LOG"=w3647:string)  [unwired: 8 in, 1 out]
                        n2601 = local write "EVENT LOG"(w3647) -> ()
                      }
                      frame #8 {
                        n2602 = Wait (ms)(milliseconds to wait=u32 50) -> ()  [unwired: 1 out]
                      }
                      frame #9 {
                        n2603 = local read "tested by"() -> (w3650:string)
                        n2604 = Concatenate Strings("Tested By :" ("Content"), w3650) -> (w3651:string)
                        n2605 = local read "EVENT LOG"() -> (w3654:string)
                        n2606 = call "Event Log.vi"("Content"=w3651, "EVENT LOG"=w3654) -> ("EVENT LOG"=w3653:string)  [unwired: 8 in, 1 out]
                        n2607 = local write "EVENT LOG"(w3653) -> ()
                      }
                      frame #10 {
                        n2608 = Wait (ms)(milliseconds to wait=u32 50) -> ()  [unwired: 1 out]
                      }
                      frame #11 {
                        n2609 = local read "TEST STANDARD"() -> (w3657:T5)
                        n2610 = case shown="\"ASTM D6079\", Default" w3657 {
                          tunnel: ["ASTM D6079" "ISO 12156" "CEC F-096-A-06" "Custom"] -> w3656
                          frame "ASTM D6079", Default {
                          }
                          frame "ISO 12156" {
                          }
                          frame "CEC F-096-A-06" {
                          }
                          frame "Custom" {
                          }
                        }
                        n2611 = Concatenate Strings("Test Standard :" ("Content"), w3656) -> (w3658:string)
                        n2612 = local read "EVENT LOG"() -> (w3661:string)
                        n2613 = call "Event Log.vi"("Content"=w3658, "EVENT LOG"=w3661) -> ("EVENT LOG"=w3660:string)  [unwired: 8 in, 1 out]
                        n2614 = local write "EVENT LOG"(w3660) -> ()
                      }
                      frame #12 {
                        n2615 = Wait (ms)(milliseconds to wait=u32 50) -> ()  [unwired: 1 out]
                      }
                      frame #13 {
                        n2616 = local read "Fuel Discription :"() -> (w3667:string)
                        n2617 = Concatenate Strings("Fuel Description :" ("Content"), w3667) -> (w3668:string)
                        n2618 = local read "EVENT LOG"() -> (w3671:string)
                        n2619 = call "Event Log.vi"("Content"=w3668, "EVENT LOG"=w3671) -> ("EVENT LOG"=w3670:string)  [unwired: 8 in, 1 out]
                        n2620 = local write "EVENT LOG"(w3670) -> ()
                      }
                      frame #14 {
                        n2621 = Wait (ms)(milliseconds to wait=u32 50) -> ()  [unwired: 1 out]
                      }
                      frame #15 {
                        n2622 = local read "Remarks :"() -> (w3673:string)
                        n2623 = Concatenate Strings("Remarks :" ("Content"), w3673) -> (w3674:string)
                        n2624 = local read "EVENT LOG"() -> (w3677:string)
                        n2625 = call "Event Log.vi"("Content"=w3674, "EVENT LOG"=w3677) -> ("EVENT LOG"=w3676:string)  [unwired: 8 in, 1 out]
                        n2626 = local write "EVENT LOG"(w3676) -> ()
                      }
